vi "GetInputCount.vi"(8 "error in (no error)":errorcluster, 11 "session id in":i32) -> (0 "error out":errorcluster, 2 "InputCount":i32, 3 "session id out":i32)   [LabVIEW 2017, in "libonnx_wrapper.lvlib"]
doc: "/**\n * @brief Получить количество входов модели\n * \n * Возвращает число входных тензоров, которые ожидает модель.\n * Большинство моделей имеют 1 вход, но некоторые (например, мульти-модальные)\n * могут иметь несколько.\n * \n * @param sessionId [IN] ID сессии\n * \n * @return int32: Количество входов (0 или больше)\n * @return int32: 0 если сессия не найдена или не загружена\n */\nint GetInputCount(int sessionId);"
uses:
  libonnx_wrapper.lvlib
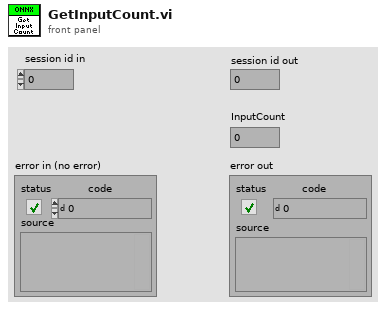
[diagram p1: front panel]
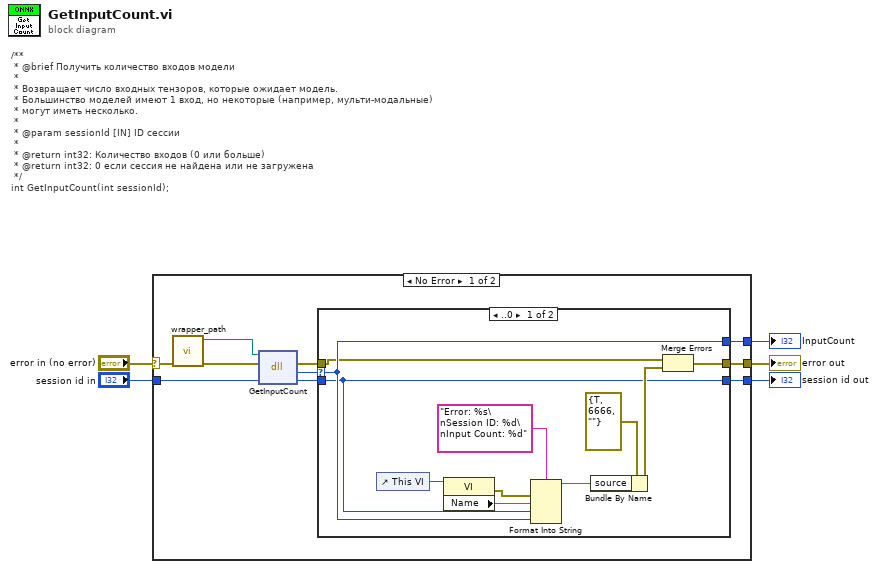
[diagram p0: block diagram]
diagram:
  # "/**\n * @brief Получить количество входов модели\n * \n * Возвращает число входных тензоров, которые ожидает модель.\n * Большинство моделей имеют 1 вход, но некоторые (например, мульти-модальные)\n * могут иметь несколько.\n * \n * @param sessionId [IN] ID сессии\n * \n * @return int32: Количество входов (0 или больше)\n * @return int32: 0 если сессия не найдена или не загружена\n */\nint GetInputCount(int sessionId);"
  n1 = case shown="No Error" "error in (no error)" {
    selector: "error in (no error)" -> [w6 w31]
    tunnel: "session id in" -> [w13 w30]
    tunnel: [w10 w31] -> w4
    tunnel: [w8 w30] -> w3
    tunnel: [w7 _] -> w2
    frame No Error {
      n2 = call "wrapper_path.vi"("error in (no error)"=w6) -> ("error out"=w15:errorcluster, "wrapper path"=w14:path)  [unwired: 9 in]
      n3 = dll-call lib="home/ivan/LabVIEWData/ONNX/Test/libonnx_wrapper/unix64/libonnx_wrapper.so" fn="GetInputCount"(path in=w14, error in=w15, "sessionId"=w13) -> (error out=w11:errorcluster, "return"=w12:i32, "sessionId"=w9:i32)  [unwired: 1 in, 1 out]
      n4 = case shown="..0" w12 {
        selector: w12 -> [w20 w27]
        tunnel: w11 -> [w16 w29]
        tunnel: [w17 w29] -> w10
        tunnel: w9 -> [w18 w28]
        tunnel: [w18 w28] -> w8
        tunnel: [w20 w27] -> w7
        frame ..0 {
          n5 = control-ref of="This VI"() -> (w23:refnum<vi>)
          n6 = property class="VI"(reference=w23) -> (error out=w19:errorcluster, "Name"=w22:string)  [unwired: 1 in, 1 out]
          n7 = Format Into String(format string="Error: %s\nSession ID: %d\nInput Count: %d", error in=w19, w22, w18, w20) -> (resulting string=w24:string)  [unwired: 1 in, 1 out]
          n8 = Bundle By Name(cluster=errorcluster {"status"=TRUE, "code"=6666, "source"=""} ("error out"), "source"=w24) -> (w25:errorcluster)
          n9 = Merge Errors(w16, w25) -> (w17:errorcluster)
        }
        frame 1.. {
        }
      }
    }
    frame Error {
    }
  }
  "error out" <- w4
  "session id out" <- w3
  "InputCount" <- w2
